vi "tx_demo.vi"() -> ()   [LabVIEW 2023]
uses:
  <vilib>/measure/NI_MABase.lvlib
  <instrlib>/niUSRP/niUSRP Write Tx Data (CDB WDT).vi
panel:
  out "Waveform Graph":waveform(dbl)(graph)
  in  "signal type":T1(ring)
  in  "frequency":dbl=10.0 format="%0.2p"
  in  "stop":bool
  in  "active antenna":string
  in  "IQ rate":dbl=100000.0 format="%#_6p"
  in  "gain":dbl format="%#_6f"
  in  "carrier frequency":dbl=100000.0 format="%#_6p"
  in  "device names":refnum<k15>
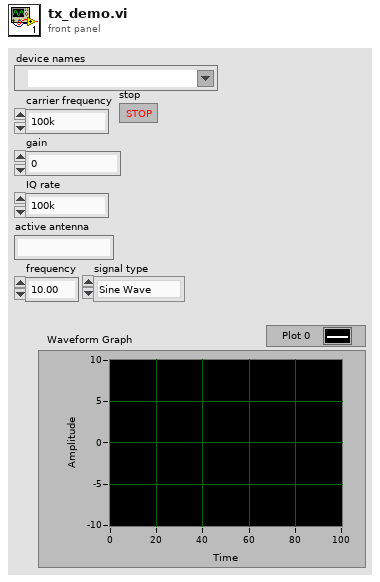
[diagram p1: front panel]
types:
  T1 = enum16{"Sine Wave", "Triangle Wave", "Square Wave", "Sawtooth Wave"}
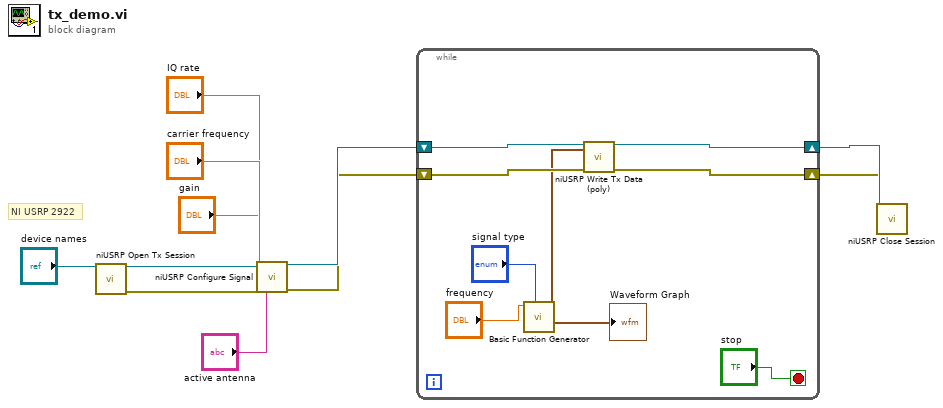
[diagram p0: block diagram]
diagram:
  # "NI USRP 2922"
  n1 = call <instrlib>:"niUSRP Open Tx Session.vi"("device names"="device names") -> ("session handle out"=w10:refnum<k15>, "error out"=w9:errorcluster)  [unwired: 13 in]
  n2 = call <instrlib>:"niUSRP Configure Signal.vi"("session handle"=w10, "IQ rate"="IQ rate", "carrier frequency"="carrier frequency", "gain"="gain", "error in (no error)"=w9, "active antenna"="active antenna") -> ("session handle out"=w8:refnum<k15>, "error out"=w7:errorcluster)  [unwired: 5 in, 3 out]
  n3 = while {
    shift-right: [w17] -> w6
    shift-left: w8 -> [w19]
    shift-right: [w16] -> w5
    shift-left: w7 -> [w18]
    stop <- "stop" stop-if-true
    n4 = call <vilib>:"Basic Function Generator.vi"("signal type"="signal type", "frequency"="frequency") -> ("signal out"=w12:waveform(dbl))  [unwired: 7 in, 2 out]
    "Waveform Graph" <- w12
    n5 = call-poly <instrlib>:"niUSRP Write Tx Data (poly).vi"("session handle"=w19, "data"=w12, "error in (no error)"=w18) -> ("session handle out"=w17:refnum<k15>, "error out"=w16:errorcluster)  [unwired: 11 in]
  }
  n6 = call <instrlib>:"niUSRP Close Session.vi"("session handle"=w6, "error in (no error)"=w5) -> ()  [unwired: 13 in, 1 out]
